vi "waveform_time_info.vi"() -> ()   [LabVIEW 2021]
panel:
  out "Waveform Graph":waveform(dbl)[](graph)
  out "Waveform Chart":waveform(dbl)[](graph)
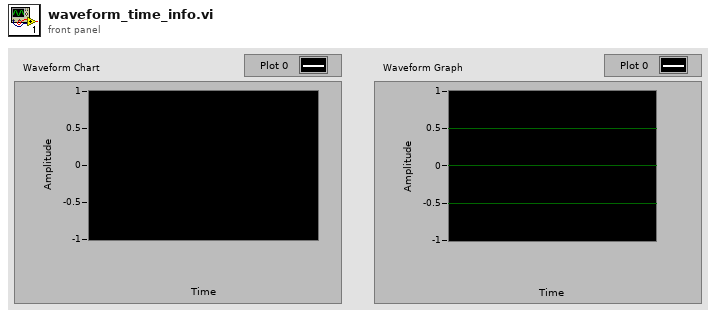
[diagram p1: front panel]
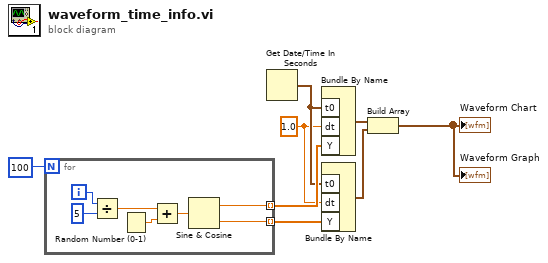
[diagram p0: block diagram]
diagram:
  w5 = 1.0 ("dt")
  n1 = for {
    N: 100 -> [_]
    tunnel: [w10] -> w7 mode=indexing
    tunnel: [w9] -> w4 mode=indexing
    i -> [w15]
    n2 = Divide(x=w15, y=5) -> (x/y=w12:dbl)
    n3 = Random Number (0-1)() -> (number: 0 to 1=w13:dbl)
    n4 = Add(x=w12, y=w13) -> (x+y=w11:dbl)
    n5 = Sine & Cosine(0:w11) -> (1:w10:dbl, 2:w9:dbl)
  }
  n6 = Get Date/Time In Seconds() -> (seconds since 1Jan1904=w6:timestamp)
  n7 = Bundle By Name("t0"=w6, "dt"=w5, "Y"=w7) -> (w3:waveform(dbl))  [unwired: 1 in]
  n8 = Bundle By Name("t0"=w6, "dt"=w5, "Y"=w4) -> (w2:waveform(dbl))  [unwired: 1 in]
  n9 = Build Array "Build Array"(w3, w2) -> (→"Waveform Graph" →"Waveform Chart":waveform(dbl)[])
